vi "Configure Output ALC State.vi"(8 "error in (no error)":errorcluster, 9 "Enable Automatic Leveling Control State (F:OFF)":bool, 10 "Platform Slot Number (10)":i16=10 min=-1 max=255, 11 "VISA resource name":refnum<visa-resource-name>) -> (0 "error out":errorcluster, 3 "VISA resource name out":refnum<visa-resource-name>)   [LabVIEW 2018, in "LTB-1.lvlib" / "3150.lvlib"]
doc: "Configures the power tracking that controls the output power level. The power tracking is done via the ALC (Automatic Leveling Control) loop. The state of the ALC loop (on or off) is used only when the POWer control mode is active.\n\n<B>Note:</B>\nThis command is applicable only for <B>Self-adjusting module</B> type of 3150. For standard module, \"Power control option not available.\" message will be returned as it doesn't support Output Power control mode. Refer IQS-3150 user manual for more information."
uses:
  3150.lvlib
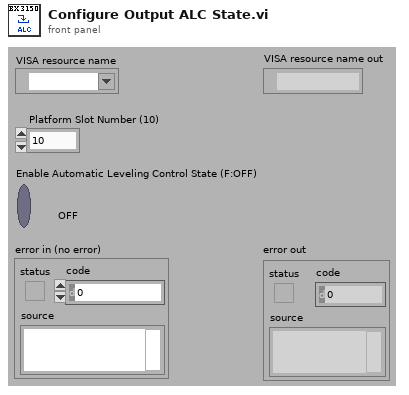
[diagram p1: front panel]
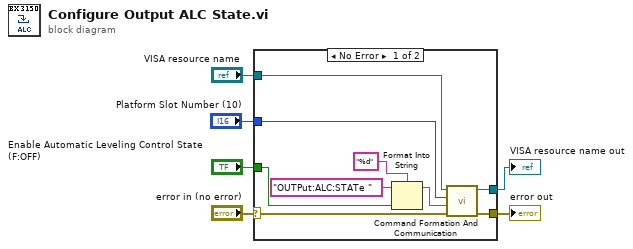
[diagram p0: block diagram]
diagram:
  n1 = case shown="No Error" "error in (no error)" {
    selector: "error in (no error)" -> [w14 w16]
    tunnel: "VISA resource name" -> [w15 w17]
    tunnel: [w13 w17] -> w4
    tunnel: [w12 w16] -> w3
    tunnel: "Enable Automatic Leveling Control State (F:OFF)" -> [w10 _]
    tunnel: "Platform Slot Number (10)" -> [w7 _]
    frame No Error {
      n2 = Format Into String(format string="%d", initial string="OUTPut:ALC:STATe " ("Command"), w10) -> (resulting string=w8:string)  [unwired: 1 in, 1 out]
      n3 = call "Command Formation And Communication.vi"("error in (no error)"=w14, "Command"=w8, "Platform Slot Number"=w7, "VISA resource name"=w15) -> ("error out"=w12:errorcluster, "VISA resource name out"=w13:refnum<visa-resource-name>)  [unwired: 1 in, 5 out]
    }
    frame Error {
    }
  }
  "VISA resource name out" <- w4
  "error out" <- w3
